vi "Create SUBSCRIBE Packet.vi"(5 "SUBSCRIBE in":refnum<class "SUBSCRIBE.lvclass">, 8 "error in (no error)":errorcluster, 9 "Packet ID (empty: Generate new)":u16 format="%04x", 11 "Topic Subscriptions":T1[](array[typedef])) -> (0 "error out":errorcluster, 3 "SUBSCRIBE out":refnum<class "SUBSCRIBE.lvclass">)   [LabVIEW 2013, in "SUBSCRIBE.lvclass"]
uses:
  SUBSCRIBE.lvclass
  Topic Subscription -- cluster.ctl
  ControlPacket/QualityOfService -- enum.ctl
  ControlPacket/ControlPacket.lvclass/ControlPacket.ctl
  ControlPacket/ControlPacket.lvclass
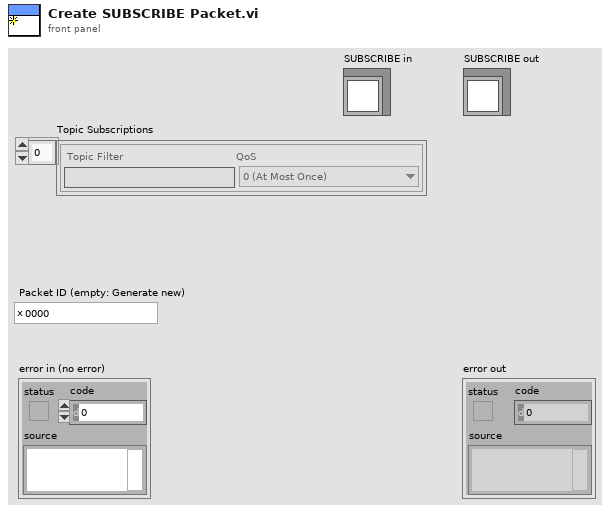
[diagram p1: front panel]
types:
  T1 = typedef "SUBSCRIBE.lvclass/Topic Subscription -- cluster.ctl" = cluster{"Topic Filter":string, "QoS":T2}
  T2 = typedef "ControlPacket.lvclass/QualityOfService -- enum.ctl" = enum16{"0 (At Most Once)", "1 (At Least Once)", "2 (Exactly Once)"}
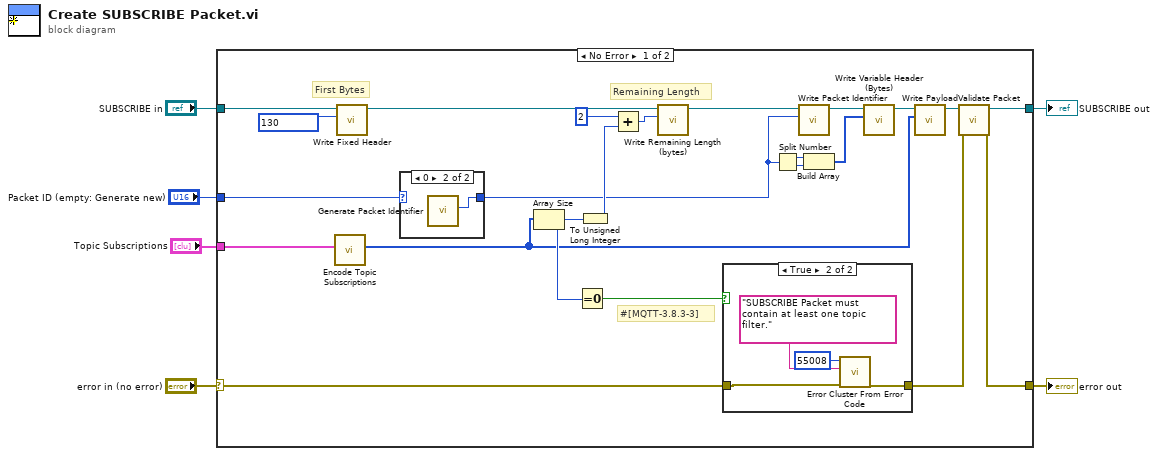
[diagram p0: block diagram]
diagram:
  n1 = case shown="No Error" "error in (no error)" {
    selector: "error in (no error)" -> [w16 w38]
    tunnel: [w11 w38] -> w3
    tunnel: [w10 w37] -> w2
    tunnel: "SUBSCRIBE in" -> [w29 w37]
    tunnel: "Packet ID (empty: Generate new)" -> [w8 _]
    tunnel: "Topic Subscriptions" -> [w14 _]
    frame No Error {
      # "#[MQTT-3.8.3-3]"
      # "Remaining Length"
      # "First Bytes"
      n2 = call "Encode Topic Subscriptions.vi"("Topic Subscriptions"=w14) -> ("Payload"=w13:u8[])  [unwired: 10 in]
      n3 = call "Write Fixed Header.vi"("Fixed Header"=u8 130, "ControlPacket in"=w29) -> ("ControlPacket out"=w28:refnum<class "SUBSCRIBE.lvclass">)  [unwired: 9 in]
      n4 = case shown="0" w8 {
        selector: w8 -> [w30 _]
        tunnel: [w30 w31] -> w7
        frame Default {
        }
        frame 0 {
          n5 = call "Generate Packet Identifier.vi"() -> ("Packet Identifier"=w31:u16)  [unwired: 11 in]
        }
      }
      n6 = Array Size(array=w13) -> (size(s)=w17:i32)
      n7 = Equal To 0?(x=w17) -> (x = 0?=w15:bool)
      n8 = To Unsigned Long Integer(number=w17) -> (unsigned 32bit integer=w18:u32)
      n9 = Add(x=u32 2 ("Remaining Length (bytes)"), y=w18) -> (x+y=w20:u32)
      n10 = call "Write Remaining Length (bytes).vi"("Remaining Length (bytes)"=w20, "ControlPacket in"=w28) -> ("ControlPacket out"=w24:refnum<class "SUBSCRIBE.lvclass">)  [unwired: 9 in]
      n11 = case shown="True" w15 {
        tunnel: w16 -> [w32 w35]
        tunnel: [w32 w36] -> w12
        frame False {
        }
        frame True {
          n12 = call <vilib>:"Error Cluster From Error Code.vi"("error in (no error)"=w35, "error message (\"\")"="SUBSCRIBE Packet must contain at least one topic filter.", "error code (0)"=55008) -> ("error out"=w36:errorcluster)  [unwired: 6 in]
        }
      }
      n13 = Split Number(x=w7) -> (hi(x)=w27:u8, lo(x)=w26:u8)
      n14 = call "Write Packet Identifier.vi"("Packet Identifier"=w7, "ControlPacket in"=w24) -> ("ControlPacket out"=w23:refnum<class "SUBSCRIBE.lvclass">)  [unwired: 9 in]
      n15 = Build Array(w27, w26) -> (w25:u8[])
      n16 = call "Write Variable Header (Bytes).vi"("Variable Header (Bytes)"=w25, "ControlPacket in"=w23) -> ("ControlPacket out"=w19:refnum<class "SUBSCRIBE.lvclass">)  [unwired: 9 in]
      n17 = call "Write Payload.vi"("Payload"=w13, "ControlPacket in"=w19) -> ("ControlPacket out"=w9:refnum<class "SUBSCRIBE.lvclass">)  [unwired: 9 in]
      n18 = call "Validate Packet.vi"("error in (no error)"=w12, "ControlPacket in"=w9) -> ("error out"=w11:errorcluster, "ControlPacket out"=w10:refnum<class "SUBSCRIBE.lvclass">)  [unwired: 8 in]
    }
    frame Error {
    }
  }
  "error out" <- w3
  "SUBSCRIBE out" <- w2
